vi "cornell-plot.vi"() -> ()   [LabVIEW 2020]
uses:
  cornell-Ktildesh2sides.ctl
  cursor action.ctl
  2Dwindow.ctl
  array action.ctl
  16981a69-1a1c-c642-ac20-7ef28ecb8088.vi
  replace cursor action stack.vi
  Q -- range multiplier -- real -- V2.vi
  Q - not nan and gtr than zero - Real.vi
  Q - not nan -- real.vi
  Q -- check range -- i -- real.vi
  array - smart min max.vi
  cornell-K0sh.vi
  cornell-K0edges.vi
  cornell-K0s.vi
  <vilib>/Comparison/Less/Less Functor/Less Functor.lvclass
panel:
  in  "parameter selectors 2":enum32{"Page 1", "Page 2"}(tab)
  in  "h/L":dbl(slide)=0.22900799999999996 min=0.0 max=0.3 step=1e-06 scale=0.0..1.0 scale format="%#_3p"
  in  "s/L":dbl(slide) min=0.0 max=0.3 step=1e-06 scale=0.0..1.0 scale format="%#_3p"
  in  "τL (sec)":dbl(slide)=10.0 min=0.0 max=0.3 step=1e-06 scale=0.0..10.0 scale format="%#_3p"
  in  "τS (sec)":dbl(slide)=3.81679389313 min=0.0 max=0.3 step=1e-12 scale=0.0..100.0 scale format="%#_3p"
  in  "parameter selectors":enum32{"Page 1"}(tab)
  in  "scale gauge: Plot: complex plane":dbl(slide)=6.232708 min=0.0 max=0.3 step=1e-06 scale=0.01..100000.0 scale format="%#_3p"
  out "Plot: sweep window":cluster{"Freq out (Hz)":dbl[], dbl[]}[](graph)
  out "Ktilde":cdb=0.005910268621655171+0.3162087805454639i format="%#_2p"
  in  "ω0 (rad/sec)":dbl(slide)=6.660846290809155 scale=0.001..10000.0 scale format="%#_2p"
  in  "parameter selectors 3":enum32{"Page 1"}(tab)
  out "Plot: vs s":cluster{dbl[], dbl[]}[](graph)
  in  "scale gauge: Plot: vs s":dbl(slide)=0.5231559999999998 min=0.0 max=0.3 step=1e-06 scale=0.01..10.0 scale format="%#_3p"
  in  "τR (sec)":dbl(slide)=0.154639 min=0.0 max=0.3 step=1e-06 scale=0.0..10.0 scale format="%#_3p"
  in  "heat link sides":T1=enum."two½"
  in  "max ω (rad/sec)":dbl(slide)=10000.00000000001 scale=0.001..5000.0
  in  "min ω (rad/sec)":dbl(slide)=0.0009999999999999994 scale=0.001..5000.0
  in  "# plot points":i64(slide)=738 scale=0.001..1500.0
  in  "# of terms in the series":i64(slide)=500 scale=0.001..1000.0
  in  "pause!":bool
  in  "go!":bool
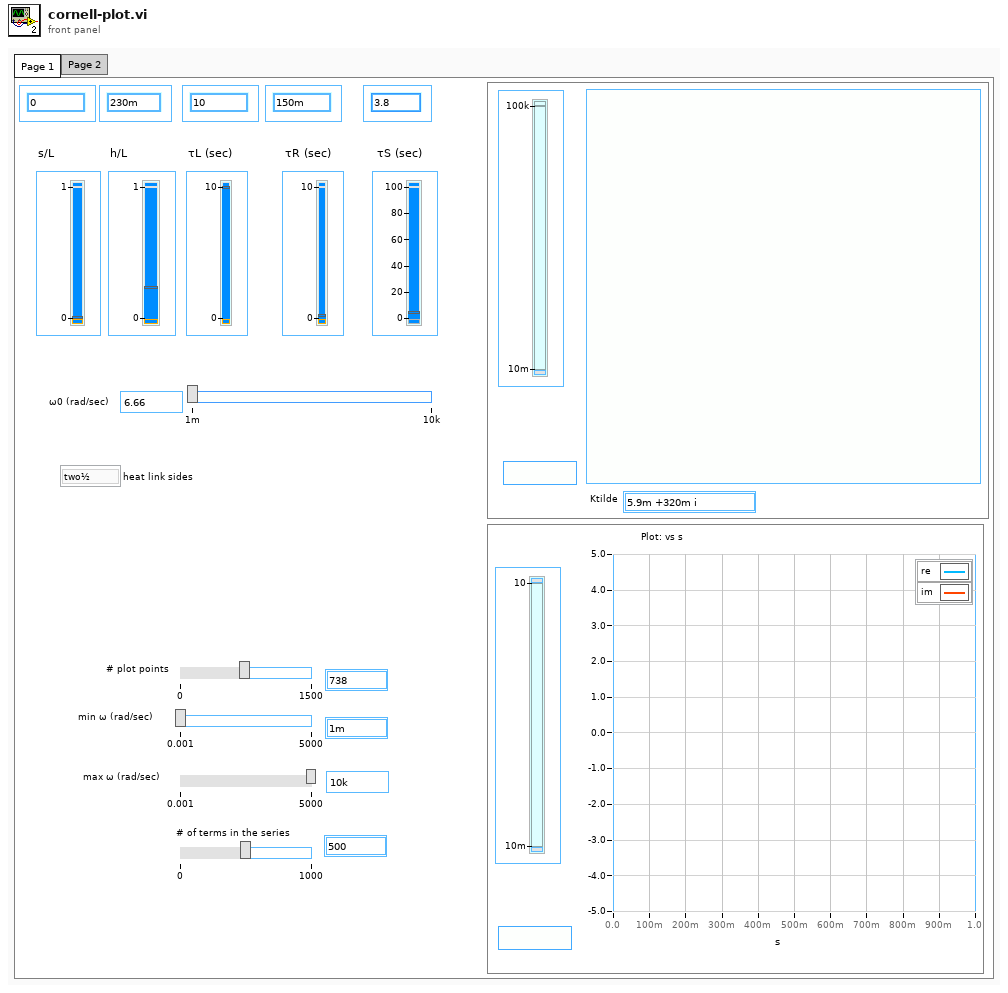
[diagram p1: front panel]
types:
  T1 = typedef "cornell-Ktildesh2sides.ctl" = enum16{"two", "one", "uni", "check1", "check2", "two½", "zcoth(z)", "z/sinh(z)", "one½", "brute"}
  T2 = typedef "2Dwindow.ctl" = cluster{"window y":dbl, "center x":dbl, "center y":dbl, "window x":dbl}
  T3 = typedef "cursor action.ctl" = enum16{"range", "read", "write", "check", "zoom out", "smart zoom out", "zoom to aspect ratio 1", "zoom to win", "zoom out 20%", "zoom in 20%", "-empty", "smart zoom out&aspect", "move range left 20%", "move range right 20%", "move range up 20%", "move range down 20%", "zoom to X win", "zoom to Y win", "zoom out X", "zoom out Y", "zoom in X", "zoom in Y", "check plot scale", "set plot color", "set Xlabel", "set Ylabel", "set cursor color"}
  T4 = typedef "array action.ctl" = enum16{"generate range", "generate log range"}
  T5 = typedef "eventvkey.ctl" = enum16{"ASCII", "Enter", "Return", "Shift", "Ctrl", "Alt", "Cmd", "Opt", "Caps", "NumLock", "Clear", "Break", "Up", "Down", "Left", "Right", "Insert", "Delete", "Home", "End", "PageUp", "PageDown", "Escape", "Help", "Pause", "ScrollLock", "F1", "F2", "F3", "F4", "F5", "F6", "F7", "F8", "F9", "F10", "F11", "F12", "F13", "F14", "F15", "F16", "F17", "F18", "F19", "F20", "F21", "F22", "F23", "F24", "Play", "VolumeUp", "VolumeDown", "Mute", "Two Byte Char"}
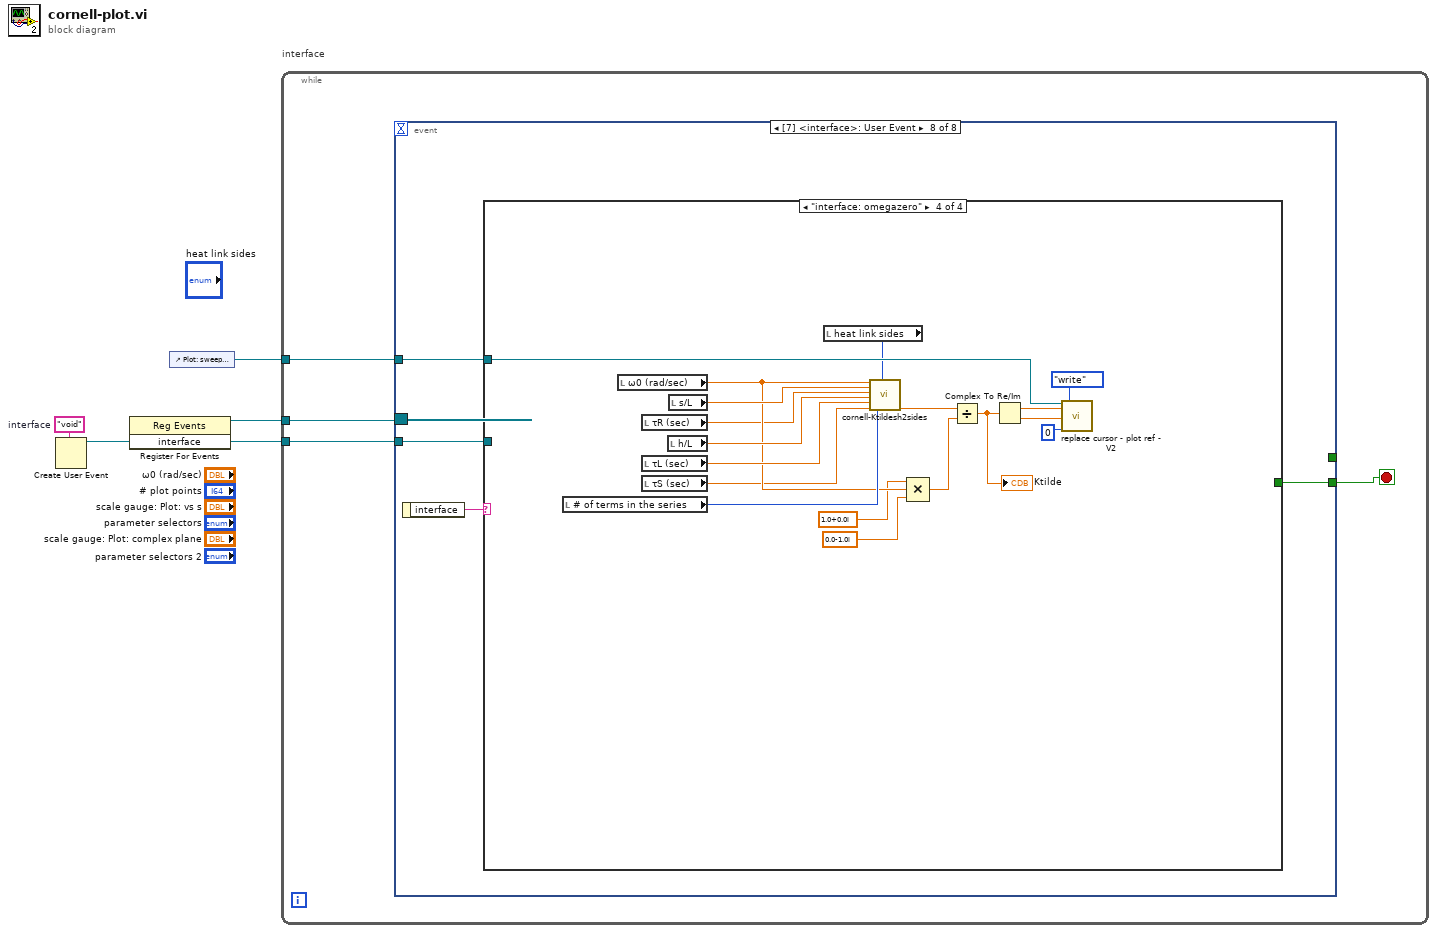
[diagram p0: block diagram]
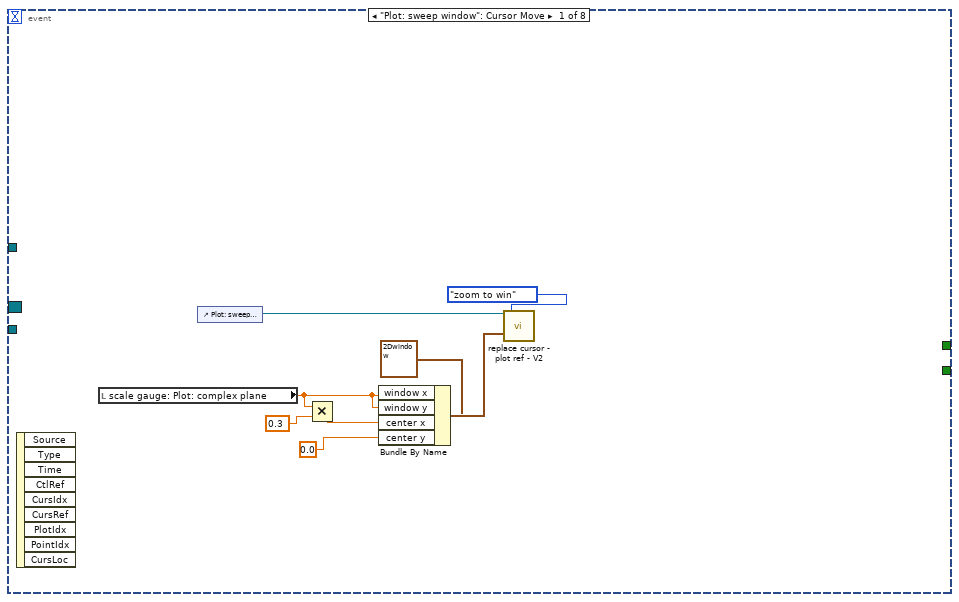
[diagram p2: hidden frame]
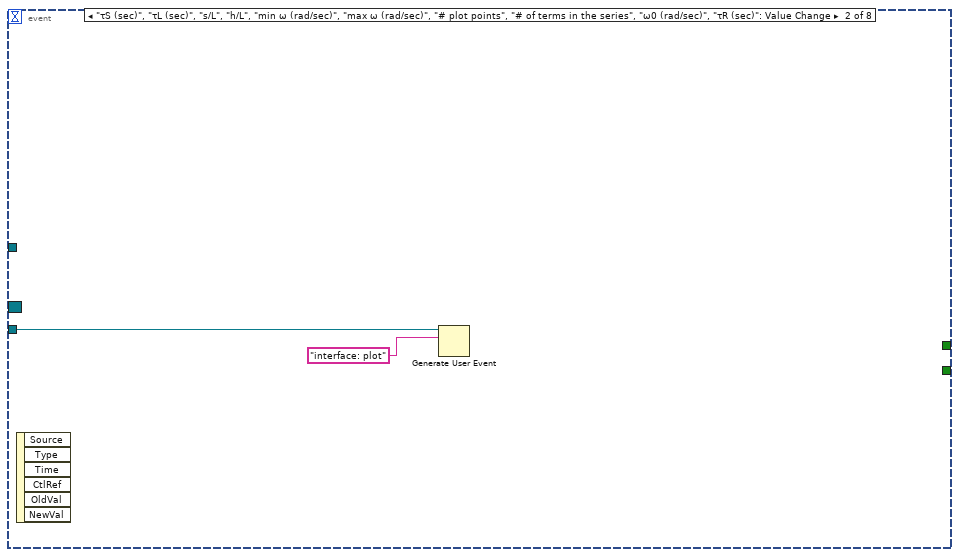
[diagram p3: hidden frame]
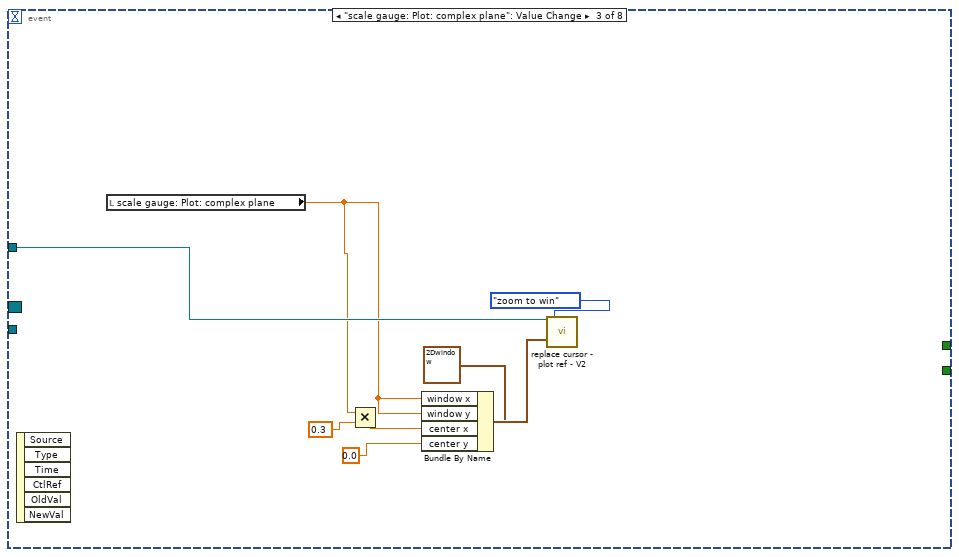
[diagram p4: hidden frame]
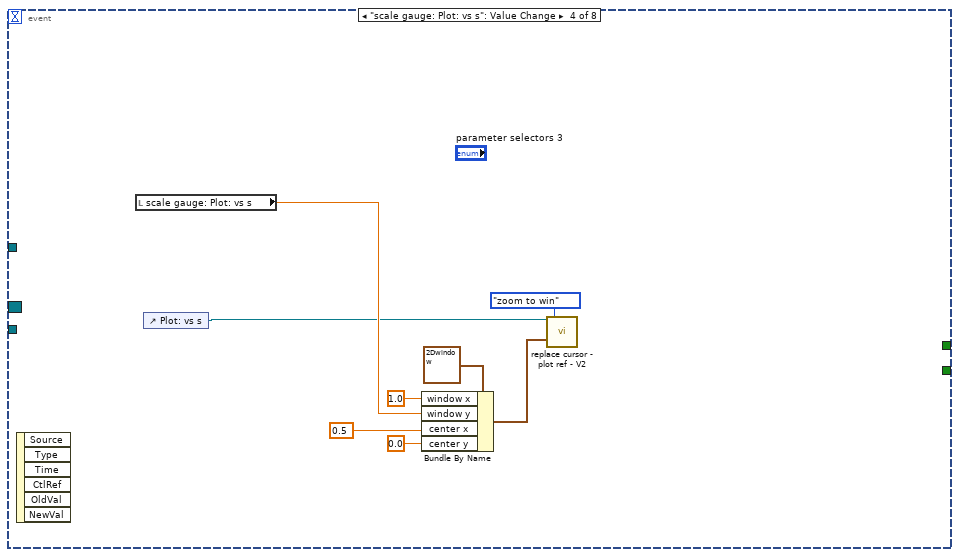
[diagram p5: hidden frame]
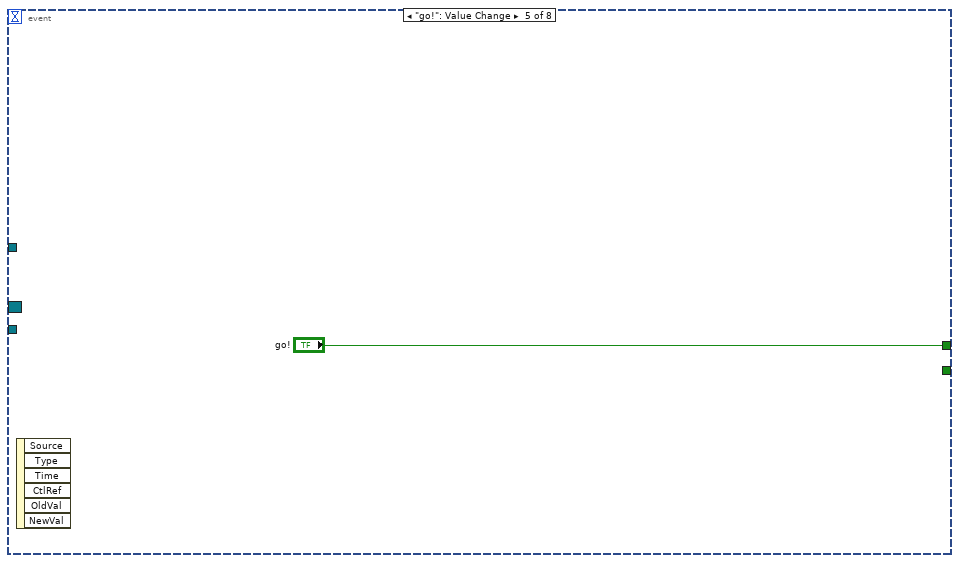
[diagram p6: hidden frame]
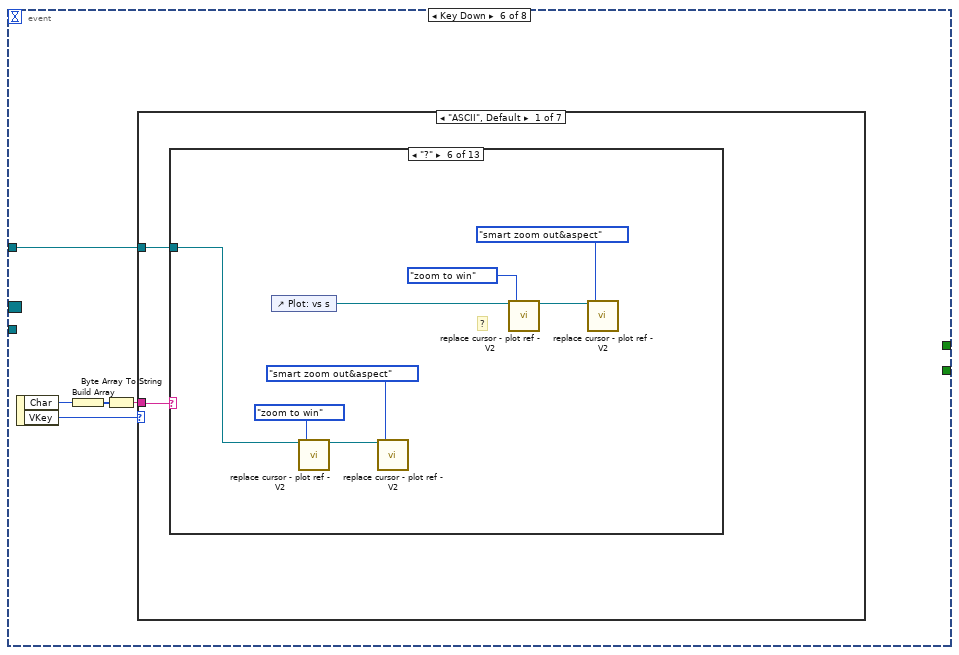
[diagram p7: hidden frame]
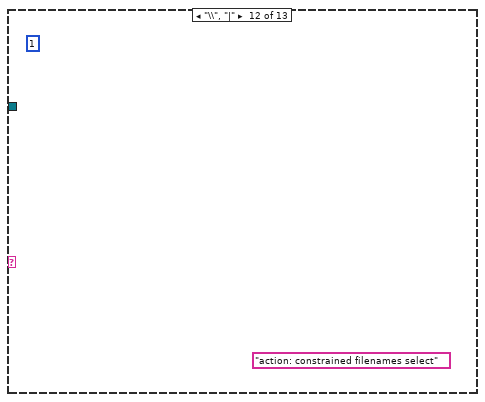
[diagram p18: hidden frame]
diagram:
  w3 = "void"  # interface
  n1 = Create User Event(user event datatype=w3) -> (user event=w1:refnum<user-event>)  [unwired: 1 in, 1 out]
  n2 = register-events(w1) -> (reference out=w4:refnum<event-registration>)  [unwired: 2 in, 1 out]
  n3 = control-ref of="Plot: sweep window"() -> (w2:refnum<vi>)
  n4 = while "interface" {
    tunnel: w4 -> [w8]
    tunnel: w2 -> [w7]
    tunnel: w1 -> [w6]
    stop <- w5 stop-if-true
    n5 = event shown="[7] <interface>: User Event" {
      selector: w8 -> [_ _ _ _ _ _ _ _]
      dyn-events: _ -> [_ _ _ _ _ _ _ _]
      timeout: _ -> [_ _ _ _ _ _ _ _]
      tunnel: [_ _ _ _ "go!" _ "pause!" _] -> _
      tunnel: w7 -> [_ _ w20 _ _ w36 _ w60]
      tunnel: w6 -> [_ w17 _ _ _ _ _ w59]
      tunnel: [_ _ _ _ _ _ _ w61] -> w5
      event "Plot: sweep window": Cursor Move {
        n6 = event-data() -> ()  [unwired: 1 in, 9 out]
        n7 = local read "scale gauge: Plot: complex plane"() -> (w15:dbl)
        n8 = control-ref of="Plot: sweep window"() -> (w14:refnum<vi>)
        n9 = Multiply(x=w15, y=0.3) -> (x*y=w16:dbl)
        n10 = Bundle By Name(cluster=T2 {"window y"=0.0021014740628288917, "center x"=44850.89441339177, "center y"=2.5658109925320947, "window x"=17480.201988350764} ("window IN"), "window x"=w15, "window y"=w15, "center x"=w16, "center y"=0.0) -> (w13:T2)
        n11 = call "replace cursor - plot ref - V2.vi"("Plot ref in"=w14, "window IN"=w13, "cursor action"=cursor_action."zoom to win") -> ()  [unwired: 13 in, 4 out]
      }
      event "τS (sec)", "τL (sec)", "s/L", "h/L", "min ω (rad/sec)", "max ω (rad/sec)", "# plot points", "# of terms in the series", "ω0 (rad/sec)", "τR (sec)": Value Change {
        n12 = event-data() -> ()  [unwired: 1 in, 6 out]
        n13 = Generate User Event(user event=w17, event data cluster="interface: plot" ("event data")) -> ()  [unwired: 2 in, 2 out]
      }
      event "scale gauge: Plot: complex plane": Value Change {
        n14 = event-data() -> ()  [unwired: 1 in, 6 out]
        n15 = local read "scale gauge: Plot: complex plane"() -> (w19:dbl)
        n16 = Multiply(x=w19, y=0.3) -> (x*y=w26:dbl)
        n17 = Bundle By Name(cluster=T2 {"window y"=0.0021014740628288917, "center x"=44850.89441339177, "center y"=2.5658109925320947, "window x"=17480.201988350764} ("window IN"), "window x"=w19, "window y"=w19, "center x"=w26, "center y"=0.0) -> (w25:T2)
        n18 = call "replace cursor - plot ref - V2.vi"("Plot ref in"=w20, "window IN"=w25, "cursor action"=cursor_action."zoom to win") -> ()  [unwired: 13 in, 4 out]
      }
      event "scale gauge: Plot: vs s": Value Change {
        n19 = event-data() -> ()  [unwired: 1 in, 6 out]
        n20 = local read "scale gauge: Plot: vs s"() -> (w30:dbl)
        n21 = control-ref of="Plot: vs s"() -> (w29:refnum<vi>)
        n22 = Bundle By Name(cluster=T2 {"window y"=0.0021014740628288917, "center x"=44850.89441339177, "center y"=2.5658109925320947, "window x"=17480.201988350764} ("window IN"), "window x"=1.0, "window y"=w30, "center x"=0.5, "center y"=0.0) -> (w34:T2)
        n23 = call "replace cursor - plot ref - V2.vi"("Plot ref in"=w29, "window IN"=w34, "cursor action"=cursor_action."zoom to win") -> ()  [unwired: 13 in, 4 out]
      }
      event "go!": Value Change {
        n24 = event-data() -> ()  [unwired: 1 in, 6 out]
      }
      event Key Down {
        n25 = event-data() -> ("Char"=w38:i16, "VKey"=w40:T5)  [unwired: 1 in]
        n26 = Build Array(w38) -> (w39:i16[])
        n27 = Byte Array To String(unsigned byte array=w39) -> (string=w37:string)
        n28 = case shown="\"ASCII\", Default" w40 {
          selector: w40 -> [_ _ _ _ _ _ w52]
          tunnel: w37 -> [w42 _ _ _ _ _ _]
          tunnel: w36 -> [w41 _ _ _ _ _ w51]
          frame "ASCII", Default {
            n29 = case shown="\"?\"" w42 {
              tunnel: w41 -> [_ _ _ _ _ w47 _ _ _ _ _ _ _]
              frame "0", Default {
              }
              frame "a" {
              }
              frame "s" {
              }
              frame "l" {
              }
              frame " " {
              }
              frame "?" {
                # "?"
                n30 = control-ref of="Plot: vs s"() -> (w43:refnum<vi>)
                n31 = call "replace cursor - plot ref - V2.vi"("Plot ref in"=w47, "cursor action"=cursor_action."zoom to win") -> ("Plot ref out"=w50:refnum<vi>)  [unwired: 14 in, 3 out]
                n32 = call "replace cursor - plot ref - V2.vi"("Plot ref in"=w50, "cursor action"=cursor_action."smart zoom out&aspect") -> ()  [unwired: 14 in, 4 out]
                n33 = call "replace cursor - plot ref - V2.vi"("Plot ref in"=w43, "cursor action"=cursor_action."zoom to win") -> ("Plot ref out"=w46:refnum<vi>)  [unwired: 14 in, 3 out]
                n34 = call "replace cursor - plot ref - V2.vi"("Plot ref in"=w46, "cursor action"=cursor_action."smart zoom out&aspect") -> ()  [unwired: 14 in, 4 out]
              }
              frame "+", ",", "-", ".", "<", "=", ">" {
              }
              frame "b" {
              }
              frame "u" {
              }
              frame "p" {
              }
              frame "q" {
              }
              frame "\\", "|" {
                (unwired) 1
                (unwired) "action: constrained filenames select" ("event data")
              }
              frame "m" {
              }
            }
          }
          frame "Escape" {
          }
          frame "PageUp" {
          }
          frame "Enter" {
          }
          frame "Caps" {
          }
          frame "PageDown" {
          }
          frame "Up".."Right" {
            n35 = case shown="\"Down\"" w52 {
              tunnel: [cursor_action."zoom in 20%" ("cursor action") cursor_action."zoom out 20%" ("cursor action") cursor_action."zoom out 20%" ("cursor action") cursor_action."zoom in 20%" ("cursor action")] -> w53
              frame "Up", Default {
              }
              frame "Down" {
              }
              frame "Left" {
              }
              frame "Right" {
              }
            }
            n36 = call "replace cursor - plot ref - V2.vi"("Plot ref in"=w51, "cursor action"=w53) -> ()  [unwired: 14 in, 4 out]
          }
        }
      }
      event "pause!": Value Change {
        n37 = event-data() -> ()  [unwired: 1 in, 6 out]
      }
      event User Event {
        n38 = event-data() -> ("interface"=w62:string)  [unwired: 1 in]
        n39 = case shown="\"interface: omegazero\"" w62 {
          tunnel: [_ _ TRUE _] -> w61
          tunnel: w60 -> [_ _ _ w135]
          tunnel: w59 -> [_ w83 _ _]
          frame "void", Default {
          }
          frame "interface: plot" {
            n40 = local read "# plot points"() -> (w78:i64)
            n41 = call "array -- generate range -- V5.vi"("action"=array_action."generate range", "ω points"=w78, "ω from"=0.0, "ω to"=1.0) -> ("ω out"=w65:dbl[])  [unwired: 7 in]
            n42 = local read "ω0 (rad/sec)"() -> (w77:dbl)
            n43 = local read "heat link sides"() -> (w63:T1)
            n44 = call "array -- generate range -- V5.vi"("action"=array_action."generate log range", "ω points"=w78, "ω from"="min ω (rad/sec)", "ω to"="max ω (rad/sec)") -> ("ω out"=w86:dbl[])  [unwired: 7 in]
            n45 = Negate(x=w86) -> (-x=w87:dbl[])
            n46 = Generate User Event(user event=w83, event data cluster="interface: omegazero" ("event data")) -> ()  [unwired: 2 in, 2 out]
            n47 = Build Array (concatenate)(w87, w86) -> (w85:dbl[])
            n48 = call "Sort 1D Array.vim"("unsorted array"=w85) -> ("sorted array"=w82:dbl[])  [unwired: 10 in]
            n49 = for {
              tunnel: w65 -> [w99] mode=indexing
              tunnel: "h/L" -> [w109]
              tunnel: "τL (sec)" -> [w108]
              tunnel: "τS (sec)" -> [w103]
              tunnel: [w106] -> w70 mode=indexing
              tunnel: "# of terms in the series" -> [w105]
              tunnel: w77 -> [w100]
              tunnel: [w99] -> w67 mode=indexing
              tunnel: "τR (sec)" -> [w98]
              tunnel: w63 -> [w97]
              n50 = call "cornell-Ktildesh2sides.vi"("ω"=w100, "s"=w99, "τGright"=w98, "h"=w109, "τGleft"=w108, "τS"=w103, "#of terms"=w105, "action"=w97) -> ("Ks(ω)"=w107:cdb)  [unwired: 11 in]
              n51 = Compound Arithmetic op=MULTIPLY(cdb 0.0-1.0i, w100, cdb 1.0+0.0i) -> (w102:cdb)
              n52 = Divide(x=w107, y=w102) -> (x/y=w106:cdb)
            }
            n53 = for {
              tunnel: w82 -> [w117] mode=indexing
              tunnel: "s/L" -> [w124]
              tunnel: "h/L" -> [w123]
              tunnel: "τL (sec)" -> [w122]
              tunnel: "τS (sec)" -> [w116]
              tunnel: [w120] -> w92 mode=indexing
              tunnel: "# of terms in the series" -> [w119]
              tunnel: "τR (sec)" -> [w113]
              tunnel: w63 -> [w112]
              n54 = call "cornell-Ktildesh2sides.vi"("ω"=w117, "s"=w124, "τGright"=w113, "h"=w123, "τGleft"=w122, "τS"=w116, "#of terms"=w119, "action"=w112) -> ("Ks(ω)"=w121:cdb)  [unwired: 11 in]
              n55 = Compound Arithmetic op=MULTIPLY(cdb 0.0-1.0i, w117, cdb 1.0+0.0i) -> (w115:cdb)
              n56 = Divide(x=w121, y=w115) -> (x/y=w120:cdb)
            }
            n57 = Complex To Re/Im(x + iy=w70) -> (x=w69:dbl[], y=w68:dbl[])
            n58 = Complex To Re/Im(x + iy=w92) -> (x=w91:dbl[], y=w90:dbl[])
            n59 = Bundle(w91, w90) -> (w89:cluster{dbl[], dbl[]})  [unwired: 1 in]
            n60 = Bundle(w67, w69) -> (w72:cluster{dbl[], dbl[]})  [unwired: 1 in]
            n61 = Bundle(w67, w68) -> (w66:cluster{dbl[], dbl[]})  [unwired: 1 in]
            n62 = disable-structure shown="Disabled" {
              frame Disabled {
                n63 = call "replace plot - plot ref - V2.vi"("cursor action"=cursor_action."write") -> ("Array X IN"=w111:dbl[])  [unwired: 14 in, 4 out]
              }
              frame Enabled {
              }
            }
            n64 = Build Array(w89) -> (→"Plot: sweep window":cluster{dbl[], dbl[]}[])
            n65 = Build Array(w72, w66) -> (→"Plot: vs s":cluster{dbl[], dbl[]}[])
          }
          frame "interface: exit" {
          }
          frame "interface: omegazero" {
            n66 = local read "# of terms in the series"() -> (w134:i64)
            n67 = local read "ω0 (rad/sec)"() -> (w131:dbl)
            n68 = local read "τR (sec)"() -> (w127:dbl)
            n69 = local read "τL (sec)"() -> (w141:dbl)
            n70 = local read "τS (sec)"() -> (w129:dbl)
            n71 = local read "h/L"() -> (w139:dbl)
            n72 = local read "s/L"() -> (w140:dbl)
            n73 = local read "heat link sides"() -> (w126:T1)
            n74 = call "cornell-Ktildesh2sides.vi"("ω"=w131, "s"=w140, "τGright"=w127, "h"=w139, "τGleft"=w141, "τS"=w129, "#of terms"=w134, "action"=w126) -> ("Ks(ω)"=w138:cdb)  [unwired: 11 in]
            n75 = Compound Arithmetic op=MULTIPLY(cdb 1.0+0.0i, w131, cdb 0.0-1.0i) -> (w130:cdb)
            n76 = Divide(x=w138, y=w130) -> (x/y=w133:cdb)
            "Ktilde" <- w133
            n77 = Complex To Re/Im(x + iy=w133) -> (x=w142:dbl, y=w143:dbl)
            n78 = call "replace cursor - plot ref - V2.vi"("Plot ref in"=w135, "new X"=w142, "new  Y"=w143, "cursor index"=0, "cursor action"=cursor_action."write") -> ()  [unwired: 11 in, 4 out]
          }
        }
      }
    }
  }
